vi "CoboltLaser_BasicWriteReadCheck.vi"(0 "ComPort":refnum<visa-resource-name>, 1 "Command":string, 2 "ResponseWaitTime (s)":dbl=0.5 min=0.0 max=100.0 step=0.1, 3 "ExpectedResponseType":T1 items=["Any", "Digits Only", "Non-Digits Only"], 4 "ExpectedResponseMinimumLength":i32 min=0 step=1, 5 "ErrorMessage":string, 6 "CheckResponse":bool=TRUE, 7 "error in (no error)":errorcluster) -> (20 "ComPortOut":refnum<visa-resource-name>, 21 "Response":string, 22 "ResponseOK":bool, 27 "error out":errorcluster)   [LabVIEW 2012, in "Cobolt.lvclass"]
doc: "Use this template to build a VI to use as a subVI."
uses:
  Template/Cobolt.lvclass
  CoboltLaser_Controls/ExpectedResponseType.ctl
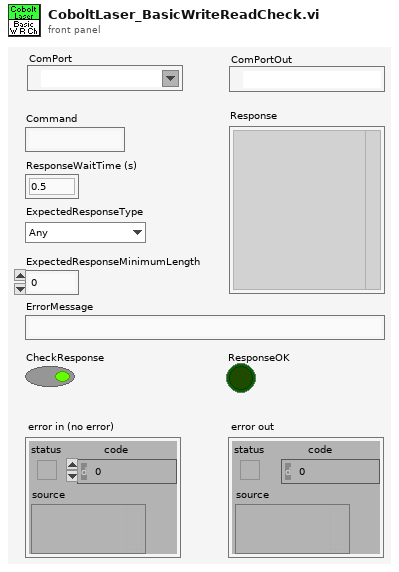
[diagram p1: front panel]
types:
  T1 = typedef "Cobolt.lvclass/ExpectedResponseType.ctl" = u16
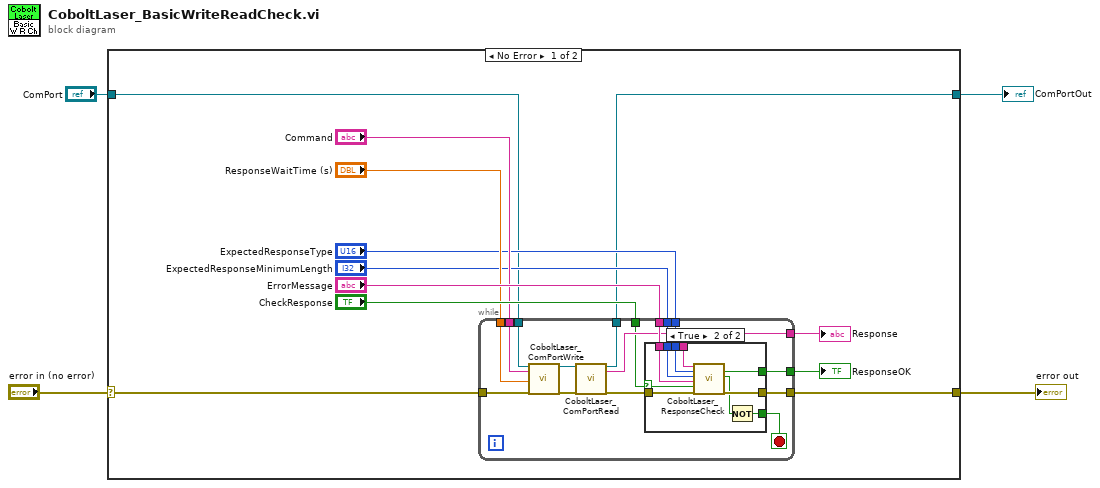
[diagram p0: block diagram]
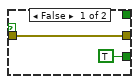
[diagram p2: hidden frame]
diagram:
  n1 = case shown="No Error" "error in (no error)" {
    selector: "error in (no error)" -> [w16 w46]
    tunnel: [w15 w46] -> w3
    tunnel: [w6 w45] -> w2
    tunnel: "ComPort" -> [w5 w45]
    frame No Error {
      n2 = while {
        tunnel: [w31] -> w6
        tunnel: [w30] -> w15
        tunnel: "CheckResponse" -> [w18]
        tunnel: w5 -> [w29]
        tunnel: [w26] -> w14
        tunnel: "Command" -> [w25]
        tunnel: w16 -> [w24]
        tunnel: "ErrorMessage" -> [w23]
        tunnel: [w19] -> w10
        tunnel: "ResponseWaitTime (s)" -> [w22]
        tunnel: "ExpectedResponseMinimumLength" -> [w20]
        tunnel: "ExpectedResponseType" -> [w21]
        stop <- w17 stop-if-true
        n3 = call "CoboltLaser_ComPortWrite.vi"("ComPort"=w29, "Command"=w25, "ResponseWaitTime (s)"=w22, "error in (no error)"=w24) -> ("ComPortOut"=w28:refnum<visa-resource-name>, "error out"=w27:errorcluster)  [unwired: 14 in]
        n4 = call "CoboltLaser_ComPortRead.vi"("ComPort"=w28, "error in (no error)"=w27) -> ("ComPort Out"=w31:refnum<visa-resource-name>, "Response"=w19:string, "error out"=w32:errorcluster)  [unwired: 15 in]
        n5 = case shown="True" w18 {
          selector: w18 -> [_ w37]
          tunnel: w32 -> [w34 w44]
          tunnel: [w34 w43] -> w30
          tunnel: [_ w42] -> w26
          tunnel: w23 -> [_ w41]
          tunnel: w21 -> [_ w40]
          tunnel: w20 -> [_ w39]
          tunnel: w19 -> [_ w38]
          tunnel: [TRUE w35] -> w17
          frame False {
          }
          frame True {
            n6 = call "CoboltLaser_ResponseCheck.vi"("Response"=w38, "ExpectedResponseType"=w40, "ExpectedResponseMinimumLength"=w39, "ErrorMessage"=w41, "GenerateErrorIfFail"=w37, "ErrorIn"=w44) -> ("ResponseOK"=w42:bool, "Retry"=w36:bool, "ErrorOut"=w43:errorcluster)  [unwired: 11 in]
            n7 = Not(x=w36) -> (.not. x?=w35:bool)
          }
        }
      }
      "Response" <- w10
      "ResponseOK" <- w14
    }
    frame Error {
    }
  }
  "error out" <- w3
  "ComPortOut" <- w2
